vi "Filter Disabled Devices from Bus by ID.vi"(8 "error in":errorcluster, 9 "BusData":T1[](array[typedef]), 10 "PCCID":T2, 11 "Generic Optimization in":refnum<class "Generic Optimization.lvclass">) -> (0 "dup error out":errorcluster, 2 "Filtered Bus by ID":T1[](array[typedef]), 3 "Generic Optimization out":refnum<class "Generic Optimization.lvclass">)   [LabVIEW 2018, in "Generic Optimization Actor.lvlib" / "Generic Optimization.lvclass"]
uses:
  Generic Optimization.lvclass
  <vilib>/ORNL/CSEISMIC DDS/CSEISMIC DDS Base/Data Types/Controls/DeviceID.ctl
  Optimization Controls/Bus by ID.ctl
  C:/Users/Administrator/Desktop/2018LabVIEW EMS/Device Communication and Control Abstract Actor/Device Communication and Control Abstract/Device Communication and Control Abstract.lvclass
  C:/Users/Administrator/Desktop/2018LabVIEW EMS/EMS Generic Actor/EMS Generic/EMS Generic.lvclass
  EMS Generic Actor/EMS Generic/EMS Generic.lvclass/EMS Generic.ctl
  <vilib>/ORNL/CSEISMIC DDS/CSEISMIC DDS Base/Data Types/IED_Status.ctl
  <vilib>/ORNL/CSEISMIC DDS/CSEISMIC DDS Base/Data Types/Controls/Timestamp.ctl
  EMS Generic Actor/EMS Generic/EMS Generic.lvclass
  <vilib>/ORNL/CSEISMIC DDS/CSEISMIC DDS Base/CSEISMIC DDS.lvclass
  Device Communication and Control Abstract Actor/Device Communication and Control Abstract/Device Communication and Control Abstract.lvclass
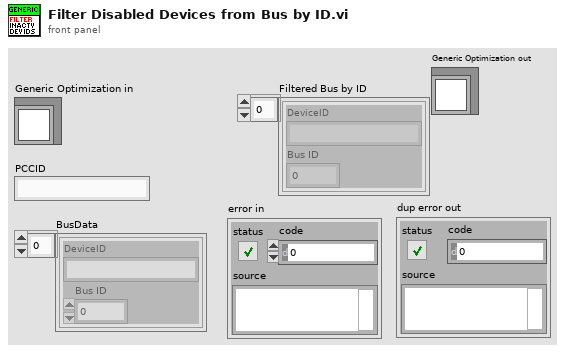
[diagram p1: front panel]
types:
  T1 = typedef "Generic Optimization Actor.lvlib/Generic Optimization.lvclass/Bus by ID.ctl" = cluster{"DeviceID":T2, "Bus ID":dbl}
  T2 = typedef "CSEISMIC DDS.lvlib/CSEISMIC DDS.lvclass/DeviceID.ctl" = string
  T3 = typedef "EMS Generic Actor.lvlib/EMS Generic.lvclass/Data Type DVRs.ctl" = cluster{"IED_Status":refnum<data-value>, "IED_Status_0":refnum<data-value>, "DER_Measurement":refnum<data-value>, "DER_Info":refnum<data-value>, "DER_Status":refnum<data-value>, "ES_Measurement":refnum<data-value>, "ES_Info":refnum<data-value>, "PV_Info":refnum<data-value>, "SmartRelay_Info":refnum<data-value>, "SmartRelay_Measurement":refnum<data-value>, "Meter_Info":refnum<data-value>, "Meter_Measurement":refnum<data-value>, "HVAC_Status":refnum<data-value>, "HVAC_Measurement":refnum<data-value>, "PriceData_RealTime":refnum<data-value>, "PriceData_Demand":refnum<data-value>, "PriceData_Energy":refnum<data-value>, "ForecastData_Long":refnum<data-value>, "ForecastData_Short":refnum<data-value>, "DER_Control":refnum<data-value>, "DER_SetPointF":refnum<data-value>, "DER_SetPointP":refnum<data-value>, "DER_SetPointQ":refnum<data-value>, "DER_SetPointPF":refnum<data-value>, "DER_SetPointV":refnum<data-value>, "PV_setCurtailment":refnum<data-value>, "PV_setRampRate":refnum<data-value>, "Relay_Control":refnum<data-value>, "Load_Control":refnum<data-value>, "HVAC_Control":refnum<data-value>, "Generator_Info":refnum<data-value>, "ForecastData_Long_Backup":refnum<data-value>, "PriceData_RealTime_Backup":refnum<data-value>}
  T4 = typedef "CSEISMIC DDS.lvlib/CSEISMIC DDS.lvclass/IED_Status.ctl" = cluster{"DeviceID":T2, "Timestamp":T5, "MicrogridID":u8, "Active":bool, "Inactive":bool, "Error":i32, "Fault":bool, "ErrorString":string}
  T5 = typedef "CSEISMIC DDS.lvlib/CSEISMIC DDS.lvclass/Timestamp.ctl" = cluster{"Seconds":u64, "Remainder":u64}
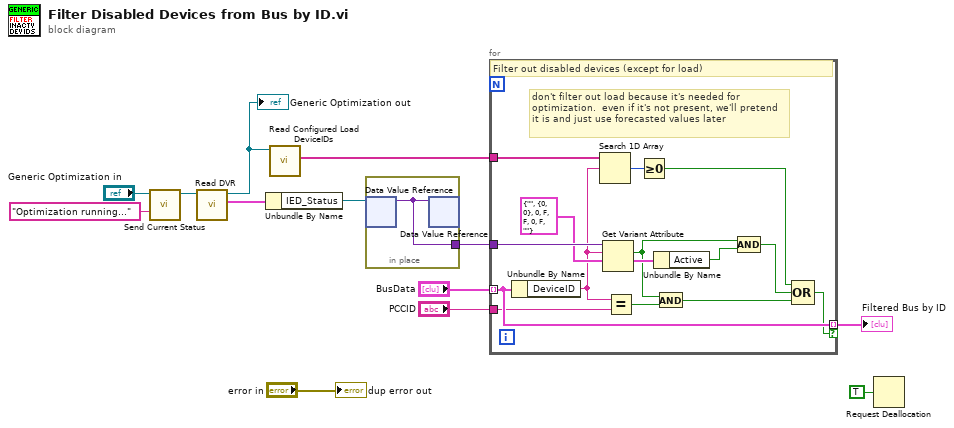
[diagram p0: block diagram]
diagram:
  n1 = call "Send Current Status.vi"("Current Status"="Optimization running...", "Device Communication and Control Abstract in"="Generic Optimization in") -> ("Device Communication and Control Abstract out"=w2:refnum<class "Generic Optimization.lvclass">)  [unwired: 8 in, 1 out]
  n2 = call "Read DVR.vi"("EMS Generic in"=w2) -> ("DVR"=w8:T3, "EMS Generic out"=w6:refnum<class "Generic Optimization.lvclass">)  [unwired: 9 in]
  "Generic Optimization out" <- w6
  n3 = Unbundle By Name(w8) -> ("IED_Status"=w10:refnum<data-value>)
  n4 = call "Read Configured Load DeviceIDs.vi"("EMS Generic in"=w6) -> ("Load DeviceIDs"=w5:T2[])  [unwired: 8 in, 2 out]
  n5 = in-place {
    in-place-border: [w14] -> w11
    n6 = in-place-dvr #1(w10) -> (w14:variant)  [unwired: 1 out]
    n7 = in-place-dvr #1(w14) -> ()  [unwired: 2 out]
  }
  n8 = for {
    tunnel: "BusData" -> [w29] mode=indexing
    tunnel: w11 -> [w22]
    tunnel: [w29] -> w12 mode=indexing if=w23
    tunnel: "PCCID" -> [w27]
    tunnel: w5 -> [w18]
    # "don't filter out load because it's needed for optimization.  even if it's not present, we'll pretend it is and just use forecasted values later"
    # "Filter out disabled devices (except for load)"
    n9 = Unbundle By Name(w29) -> ("DeviceID"=w17:T2)
    n10 = Search 1D Array(1D array=w18, element=w17) -> (index of element=w16:i32)  [unwired: 1 in]
    n11 = Get Variant Attribute(Variant=w22, name=w17, default value (empty Variant)=T4 {"DeviceID"="", "Timestamp"={"Seconds"=0, "Remainder"=0}, "MicrogridID"=0, "Active"=FALSE, "Inactive"=FALSE, "Error"=0, "Fault"=FALSE, "ErrorString"=""} ("IED_Status")) -> (found=w19:bool, value=w20:T4)  [unwired: 1 in, 2 out]
    n12 = Equal?(x=w17, y=w27) -> (x = y?=w26:bool)
    n13 = Greater Or Equal To 0?(x=w16) -> (x >= 0?=w15:bool)
    n14 = Unbundle By Name(w20) -> ("Active"=w28:bool)
    n15 = And(x=w19, y=w26) -> (x .and. y?=w24:bool)
    n16 = Compound Arithmetic op=AND(w19, w28) -> (w25:bool)
    n17 = Compound Arithmetic op=OR(w15, w25, w24) -> (w23:bool)
  }
  "Filtered Bus by ID" <- w12
  n18 = Request Deallocation(TRUE ("flag")) -> ()
  "dup error out" <- "error in"
